vi "Server Cmd Parser - Set Corrections.vi"(8 "error in":errorcluster, 10 "client request":T1={"info data"="", "answer handle"=-1}, 11 "session in":T2={"adc"={"niScope"={"channel cfg"=[], "sessions"=[], "multi cards"=FALSE, "channels"=0, "type"=enum."n/a", "memory [B/chn]"=0, "ext. clock [Hz]"=0.0, "samples count"=0, "use streaming"=FALSE, "proc setup"={"packet size [smpl]"=0, "current timeout [s]"=0.0, "blk2blk timeout [s]"=0.0, "event time"=timestamp(0 s since 1904-01-01), "temp sampl T [s]"=0.0, "data queue"=refnum, "stop notifier"=refnum, "proc ref"=refnum}, "sample width [B]"=0, "ranges [V]"=[], "trigger setup"={"coupling"=1, "level [V]"=0.0, "slope"=0, "mode"=enum."Immediate"}, "fs [Hz]"=0.0, "bitres [bit]"=0}, "3458A"={"channels"=[], "sync unit"={"VISA"="", "type"=enum."Picotest U6200A"}, "awg unit"={"type"=enum."Agilent 331xxA to 332xxA", "VISA"="", "enable 10MHz ref"=FALSE}, "sync mode"=enum."MASTER-SLAVE, MASTER clocked by TIMER", "streaming mode"=FALSE, "idn mode"=enum."Auto", "sampling mode"=enum."DCV", "Ts [s]"=0.0, "sample memory [B]"=0, "proc setup"={"channel id"=0, "packet size [smpl]"=0, "current timeout [s]"=0.0, "blk2blk timeout [s]"=0.0, "event time"=timestamp(0 s since 1904-01-01), "stop notifier"=refnum, "data queues"=[], "proc refs"=[], "bus semaphore"=refnum}, "sample size [B]"=0, "sample count"=0, "aux data"={"channel id"=0, "valid?"=[], "gain [V]"=[], "timestamp [s]"=[], "Ts [s]"=0.0, "abs timestamp"=timestamp(0 s since 1904-01-01), "t [deg C]"=[]}, "ranges [V]"=[], "aperture [s]"=0.0, "LEVEL trigger"={"edge"=enum."POS", "level [V]"=0.0, "coupling"=enum."DC"}, "trigger mode"=enum."AUTO", "measure temp.?"=FALSE, "disp mesages"=[], "shared bus?"=FALSE, "disable display?"=FALSE, "aper mode"=enum."Manual", "aper rules"=[]}, "dsdll"={"dsdll"={"dsdll path"=path "", "dsdll handle"=[], "output devices"=[], "capture devices"=[]}, "channels"=0, "device id"=0, "channel idns"=[], "proc setup"={"packet size [smpl]"=0, "current timeout [s]"=0.0, "blk2blk timeout [s]"=0.0, "event time"=timestamp(0 s since 1904-01-01), "data queue"=refnum, "stop notifier"=refnum, "proc ref"=refnum}, "samples count"=0, "fs [Hz]"=0.0}, "type"=enum."niScope", "channel idn str"=[], "aux instr idn str"=[], "modified?"=FALSE, "simadc"={"channels"=[], "range [V]"=0.0, "Ts step [s]"=0.0, "time [s]"=0.0, "fs [Hz]"=0.0, "count"=0, "smpl offset"=0, "set count"=0, "bit res"=0}, "force rst?"=FALSE, "exit mode"=enum."Immediate reset", "exit dly"=0.0, "exit tmr"=timestamp(0 s since 1904-01-01), "busy?"=FALSE, "accessed?"=FALSE, "QuADC session"={"channel cfg"=[], "sessions"=[], "multi cards"=FALSE, "channels"=0, "type"=enum."n/a", "memory [B/chn]"=0, "ext. clock [Hz]"=0.0, "samples count"=0, "use streaming"=FALSE, "proc setup"={"packet size [smpl]"=0, "current timeout [s]"=0.0, "blk2blk timeout [s]"=0.0, "event time"=timestamp(0 s since 1904-01-01), "temp sampl T [s]"=0.0, "data queue"=refnum, "stop notifier"=refnum, "proc ref"=refnum}, "sample width [B]"=0, "ranges [V]"=[], "trigger setup"={"coupling"=1, "level [V]"=0.0, "slope"=0, "mode"=enum."Immediate"}, "fs [Hz]"=0.0, "bitres [bit]"=0}}, "sequence"=[], "sequence setup"={"group setups"=[], "average cycles"=0, "range mode"=enum."Keep defaults", "fs mode"=enum."Frequency", "rng even"=0.0, "rng odd"=0.0, "folder"=path "", "name base"="", "meas id"=0, "settle [s]"=0.0}, "golpi"=refnum, "processing setup"={"mode"=enum."Raw", "call after avgs?"=FALSE, "calculate?"=FALSE, "raw mode"={"command"="", "result mode"=enum."Display console output (only Octave)", "res variable"=""}, "QWTB"={"QWTB path"=path "", "alg filter path"="", "alg ids"=[], "alg parameters"=[], "parsed parameters"=[], "selected alg id"="", "selected unc mode"=enum."None", "qwtb mcc"=100, "qwtb timeout"=90, "qwtb covg"=95.0, "qwtb ofs"=0, "qwtb lim data"=0, "multicore"={"jobs folder"=path "", "cores"=0, "max jobs"=0, "mode"=enum."Singlecore"}, "unc once?"=FALSE}}, "corrections"={"transducers"={"channels"=[], "last path"=path ""}, "digitizer"={"last path"=path "", "channel paths"=[], "channel idns"=[], "correction name"="", "channel names"=[], "folders to copy"=[], "channel valid"=[], "correction path"=path "", "correction rel path"="", "rel folders to copy"=[]}}, "assist cfg"={"P"=0, "Q"=0, "rel shift"=0.0, "ref freq"=0.0, "min fs"=0.0, "max fs tol"=0.0, "min int"=0.0, "max int"=0.0, "max err"=0.0, "max timeout"=0.0}} {"corrections"."transducers"."channels"."Phase index" min=1 step=1; "adc"."QuADC session"."trigger setup"."level [V]" format="%.2f"; "adc"."QuADC session"."trigger setup"."coupling" items=["AC"=0, "DC"=1, "HF Reject"=3, "LF Reject"=4, "AC Plus HF Reject"=1001]; "adc"."QuADC session"."channel cfg"."Clock fr. (Hz)" min=0.0 format="%#_9p"; "adc"."QuADC session"."channel cfg"."Number of JJ" min=1; "adc"."QuADC session"."channel cfg"."Range [Vpk]" min=0.0; "adc"."QuADC session"."channel cfg"."Channel" min=0; "adc"."3458A"."channels"."Range [Vpk]" min=0.0; "adc"."niScope"."trigger setup"."level [V]" format="%.2f"; "adc"."niScope"."trigger setup"."coupling" items=["AC"=0, "DC"=1, "HF Reject"=3, "LF Reject"=4, "AC Plus HF Reject"=1001]; "adc"."niScope"."channel cfg"."Range [Vpk]" min=0.0; "adc"."niScope"."channel cfg"."Channel" min=0}) -> (0 "error out":errorcluster, 3 "session out":T2={"adc"={"niScope"={"channel cfg"=[], "sessions"=[], "multi cards"=FALSE, "channels"=0, "type"=enum."n/a", "memory [B/chn]"=0, "ext. clock [Hz]"=0.0, "samples count"=0, "use streaming"=FALSE, "proc setup"={"packet size [smpl]"=0, "current timeout [s]"=0.0, "blk2blk timeout [s]"=0.0, "event time"=timestamp(0 s since 1904-01-01), "temp sampl T [s]"=0.0, "data queue"=refnum, "stop notifier"=refnum, "proc ref"=refnum}, "sample width [B]"=0, "ranges [V]"=[], "trigger setup"={"coupling"=1, "level [V]"=0.0, "slope"=0, "mode"=enum."Immediate"}, "fs [Hz]"=0.0, "bitres [bit]"=0}, "3458A"={"channels"=[], "sync unit"={"VISA"="", "type"=enum."Picotest U6200A"}, "awg unit"={"type"=enum."Agilent 331xxA to 332xxA", "VISA"="", "enable 10MHz ref"=FALSE}, "sync mode"=enum."MASTER-SLAVE, MASTER clocked by TIMER", "streaming mode"=FALSE, "idn mode"=enum."Auto", "sampling mode"=enum."DCV", "Ts [s]"=0.0, "sample memory [B]"=0, "proc setup"={"channel id"=0, "packet size [smpl]"=0, "current timeout [s]"=0.0, "blk2blk timeout [s]"=0.0, "event time"=timestamp(0 s since 1904-01-01), "stop notifier"=refnum, "data queues"=[], "proc refs"=[], "bus semaphore"=refnum}, "sample size [B]"=0, "sample count"=0, "aux data"={"channel id"=0, "valid?"=[], "gain [V]"=[], "timestamp [s]"=[], "Ts [s]"=0.0, "abs timestamp"=timestamp(0 s since 1904-01-01), "t [deg C]"=[]}, "ranges [V]"=[], "aperture [s]"=0.0, "LEVEL trigger"={"edge"=enum."POS", "level [V]"=0.0, "coupling"=enum."DC"}, "trigger mode"=enum."AUTO", "measure temp.?"=FALSE, "disp mesages"=[], "shared bus?"=FALSE, "disable display?"=FALSE, "aper mode"=enum."Manual", "aper rules"=[]}, "dsdll"={"dsdll"={"dsdll path"=path "", "dsdll handle"=[], "output devices"=[], "capture devices"=[]}, "channels"=0, "device id"=0, "channel idns"=[], "proc setup"={"packet size [smpl]"=0, "current timeout [s]"=0.0, "blk2blk timeout [s]"=0.0, "event time"=timestamp(0 s since 1904-01-01), "data queue"=refnum, "stop notifier"=refnum, "proc ref"=refnum}, "samples count"=0, "fs [Hz]"=0.0}, "type"=enum."niScope", "channel idn str"=[], "aux instr idn str"=[], "modified?"=FALSE, "simadc"={"channels"=[], "range [V]"=0.0, "Ts step [s]"=0.0, "time [s]"=0.0, "fs [Hz]"=0.0, "count"=0, "smpl offset"=0, "set count"=0, "bit res"=0}, "force rst?"=FALSE, "exit mode"=enum."Immediate reset", "exit dly"=0.0, "exit tmr"=timestamp(0 s since 1904-01-01), "busy?"=FALSE, "accessed?"=FALSE, "QuADC session"={"channel cfg"=[], "sessions"=[], "multi cards"=FALSE, "channels"=0, "type"=enum."n/a", "memory [B/chn]"=0, "ext. clock [Hz]"=0.0, "samples count"=0, "use streaming"=FALSE, "proc setup"={"packet size [smpl]"=0, "current timeout [s]"=0.0, "blk2blk timeout [s]"=0.0, "event time"=timestamp(0 s since 1904-01-01), "temp sampl T [s]"=0.0, "data queue"=refnum, "stop notifier"=refnum, "proc ref"=refnum}, "sample width [B]"=0, "ranges [V]"=[], "trigger setup"={"coupling"=1, "level [V]"=0.0, "slope"=0, "mode"=enum."Immediate"}, "fs [Hz]"=0.0, "bitres [bit]"=0}}, "sequence"=[], "sequence setup"={"group setups"=[], "average cycles"=0, "range mode"=enum."Keep defaults", "fs mode"=enum."Frequency", "rng even"=0.0, "rng odd"=0.0, "folder"=path "", "name base"="", "meas id"=0, "settle [s]"=0.0}, "golpi"=refnum, "processing setup"={"mode"=enum."Raw", "call after avgs?"=FALSE, "calculate?"=FALSE, "raw mode"={"command"="", "result mode"=enum."Display console output (only Octave)", "res variable"=""}, "QWTB"={"QWTB path"=path "", "alg filter path"="", "alg ids"=[], "alg parameters"=[], "parsed parameters"=[], "selected alg id"="", "selected unc mode"=enum."None", "qwtb mcc"=100, "qwtb timeout"=90, "qwtb covg"=95.0, "qwtb ofs"=0, "qwtb lim data"=0, "multicore"={"jobs folder"=path "", "cores"=0, "max jobs"=0, "mode"=enum."Singlecore"}, "unc once?"=FALSE}}, "corrections"={"transducers"={"channels"=[], "last path"=path ""}, "digitizer"={"last path"=path "", "channel paths"=[], "channel idns"=[], "correction name"="", "channel names"=[], "folders to copy"=[], "channel valid"=[], "correction path"=path "", "correction rel path"="", "rel folders to copy"=[]}}, "assist cfg"={"P"=0, "Q"=0, "rel shift"=0.0, "ref freq"=0.0, "min fs"=0.0, "max fs tol"=0.0, "min int"=0.0, "max int"=0.0, "max err"=0.0, "max timeout"=0.0}} {"corrections"."transducers"."channels"."Phase index" min=1 step=1; "adc"."QuADC session"."trigger setup"."level [V]" format="%.2f"; "adc"."QuADC session"."trigger setup"."coupling" items=["AC"=0, "DC"=1, "HF Reject"=3, "LF Reject"=4, "AC Plus HF Reject"=1001]; "adc"."QuADC session"."channel cfg"."Clock fr. (Hz)" min=0.0 format="%#_9p"; "adc"."QuADC session"."channel cfg"."Number of JJ" min=1; "adc"."QuADC session"."channel cfg"."Range [Vpk]" min=0.0; "adc"."QuADC session"."channel cfg"."Channel" min=0; "adc"."3458A"."channels"."Range [Vpk]" min=0.0; "adc"."niScope"."trigger setup"."level [V]" format="%.2f"; "adc"."niScope"."trigger setup"."coupling" items=["AC"=0, "DC"=1, "HF Reject"=3, "LF Reject"=4, "AC Plus HF Reject"=1001]; "adc"."niScope"."channel cfg"."Range [Vpk]" min=0.0; "adc"."niScope"."channel cfg"."Channel" min=0})   [LabVIEW 2018]
doc: "Parses Server command \"Set corrections\" and assigns the parsed parameters to the measurement session."
uses:
  measure/Meas Session.ctl
  adc/ADC Session.ctl
  drivers/niScope/niScope Session.ctl
  drivers/niScope/niScope Virtual Channel Config.ctl
  drivers/niScope/niScope Virtual Channel Mode.ctl
  drivers/niScope/niScope Virtual Channel Input Z.ctl
  drivers/niScope/niScope Virtual Channel Coupling.ctl
  drivers/niScope/niScope Type.ctl
  drivers/niScope/niScope Digitizing Process Options.ctl
  drivers/niScope/niScope Data Packet.ctl
  drivers/niScope/niScope Trigger Setup.ctl
  <instrlib>/niScope/Controls/niScope trigger coupling.ctl
  <instrlib>/niScope/Controls/niScope trigger slope.ctl
  drivers/DMM/3458A Digitizer Session.ctl
  drivers/DMM/3458A Virtual Channel Config.ctl
  drivers/Counter/Counter Session.ctl
  drivers/Counter/Counter Type.ctl
  drivers/AWG/AWG Session.ctl
  drivers/AWG/AWG Type.ctl
  drivers/DMM/3458A Sync Mode.ctl
  drivers/DMM/3458A Idn Mode.ctl
  drivers/DMM/3458A Digitizing Low Levels/Configure/Sampling Mode.ctl
  drivers/DMM/3458A Digitizing Process Options.ctl
  drivers/DMM/3458A Data Packet.ctl
  drivers/DMM/3458A Aux Record Data.ctl
  drivers/DMM/3458A Digitizing Low Levels/Configure/Level Setup.ctl
  drivers/DMM/3458A Digitizing Low Levels/Configure/First Sample Trigger.ctl
  drivers/DMM/3458A Aperture Selection Mode.ctl
  drivers/dsdll/DSDLL Session.ctl
  drivers/dsdll/dsdll source distribution/dsdll_instance.ctl
  drivers/dsdll/dsdll source distribution/dsdll_device_record.ctl
  drivers/dsdll/DSDLL Process Config.ctl
  drivers/dsdll/DSDLL Data Packet.ctl
  adc/ADC Type.ctl
  drivers/simulated_adc/SimAdc Config.ctl
  drivers/simulated_adc/SimAdc Channel Cfg.ctl
  adc/ADC On Close Action.ctl
  drivers/Quatsch_driver/QuADCDriver/QuADC Session.ctl
  drivers/Quatsch_driver/QuADCDriver/QuADC Virtual Channel Config.ctl
  drivers/Quatsch_driver/QuADCDriver/QuADC Virtual Channel Mode.ctl
  drivers/Quatsch_driver/QuADCDriver/QuADC Virtual Channel Input Z.ctl
  drivers/Quatsch_driver/QuADCDriver/QuADC Virtual Channel Coupling.ctl
  drivers/Quatsch_driver/QuADCDriver/QuADC Type.ctl
  drivers/Quatsch_driver/QuADCDriver/QuADC Digitizing Process Options.ctl
  drivers/Quatsch_driver/QuADCDriver/QuADC Data Packet.ctl
  drivers/Quatsch_driver/QuADCDriver/QuADC Trigger Setup.ctl
  measure/Meas Sequence Item.ctl
  measure/Meas Sampling Configuration.ctl
  adc/ADC Trig Config.ctl
  adc/ADC Trig Mode Source.ctl
  adc/ADC Trig Coupling.ctl
  adc/ADC Trig Slope.ctl
  measure/processing/QWTB/Meas Proc QWTB Algorithm Parameter Data.ctl
  measure/Meas Sequence Configuration.ctl
  measure/Meas Range Mode.ctl
  measure/Meas Sampling Rate Mode.ctl
  octave/golpi/mpc/golpi_session_ref.ctl
  octave/golpi/mpc/golpi_session.ctl
  octave/golpi/GOLPI Library.lvlibp/Public/GOLPI reference Type Def.ctl
  octave/golpi/GOLPI Library.lvlibp/LV Process source distribution/Pipe Handle.ctl
  measure/processing/Meas Process Config.ctl
  measure/processing/Meas Process Mode.ctl
  measure/processing/Meas Process Raw Config.ctl
  measure/processing/Meas Process Raw Result Mode.ctl
  measure/processing/QWTB/Meas Proc QWTB Setup.ctl
  measure/processing/QWTB/Meas Proc QWTB Uncertainty Mode.ctl
  measure/processing/QWTB/Meas Proc QWTB Multicore Setup.ctl
  measure/processing/QWTB/Meas Proc QWTB Multicore Type.ctl
  measure/Corrections/Corr Setup.ctl
  measure/Corrections/Corr Tranducer Item.ctl
  measure/Corrections/Corr Digitizers.ctl
  measure/Assist/Assist Panel Setup.ctl
  Server Client Request.ctl
  octave/infolib.lvlibp/Private/Get matrix polymorph parts/Get 1D String.vi
  octave/infolib.lvlibp/Private/Get matrix polymorph parts/Get 1D I64.vi
  octave/infolib.lvlibp/Private/Get key polymorph parts/GetString.vi
  octave/infolib.lvlibp
  drivers/niScope/niScope Virtual Digitizer.lvlib
  drivers/DMM/3458A Virtual Digitizer.lvlib
  drivers/Counter/Counter.lvlib
  drivers/AWG/AWG.lvlib
  drivers/DMM/3458A Digitizing Low Levels/3458A Digitizing Low Levels.lvlib
  drivers/dsdll/DSDLL Virtual Digitizer.lvlib
  octave/golpi/GOLPI Library.lvlibp/LV Process source distribution/LV Process library.lvlib
  octave/golpi/GOLPI Library.lvlibp
  octave/golpi/mpc/GOLPI Multi Process.lvlib
  drivers/Quatsch_driver/QuADCDriver/QuADC Virtual Digitizer.lvlib
  drivers/dsdll/dsdll source distribution/dsdll.lvlib
panel:
  # "ADC:"
  # "IP Address"
  # "."
  # "."
  # "."
  # ":"
  # "ADC:"
  # "IP Address"
  # "."
  # "."
  # "."
  # ":"
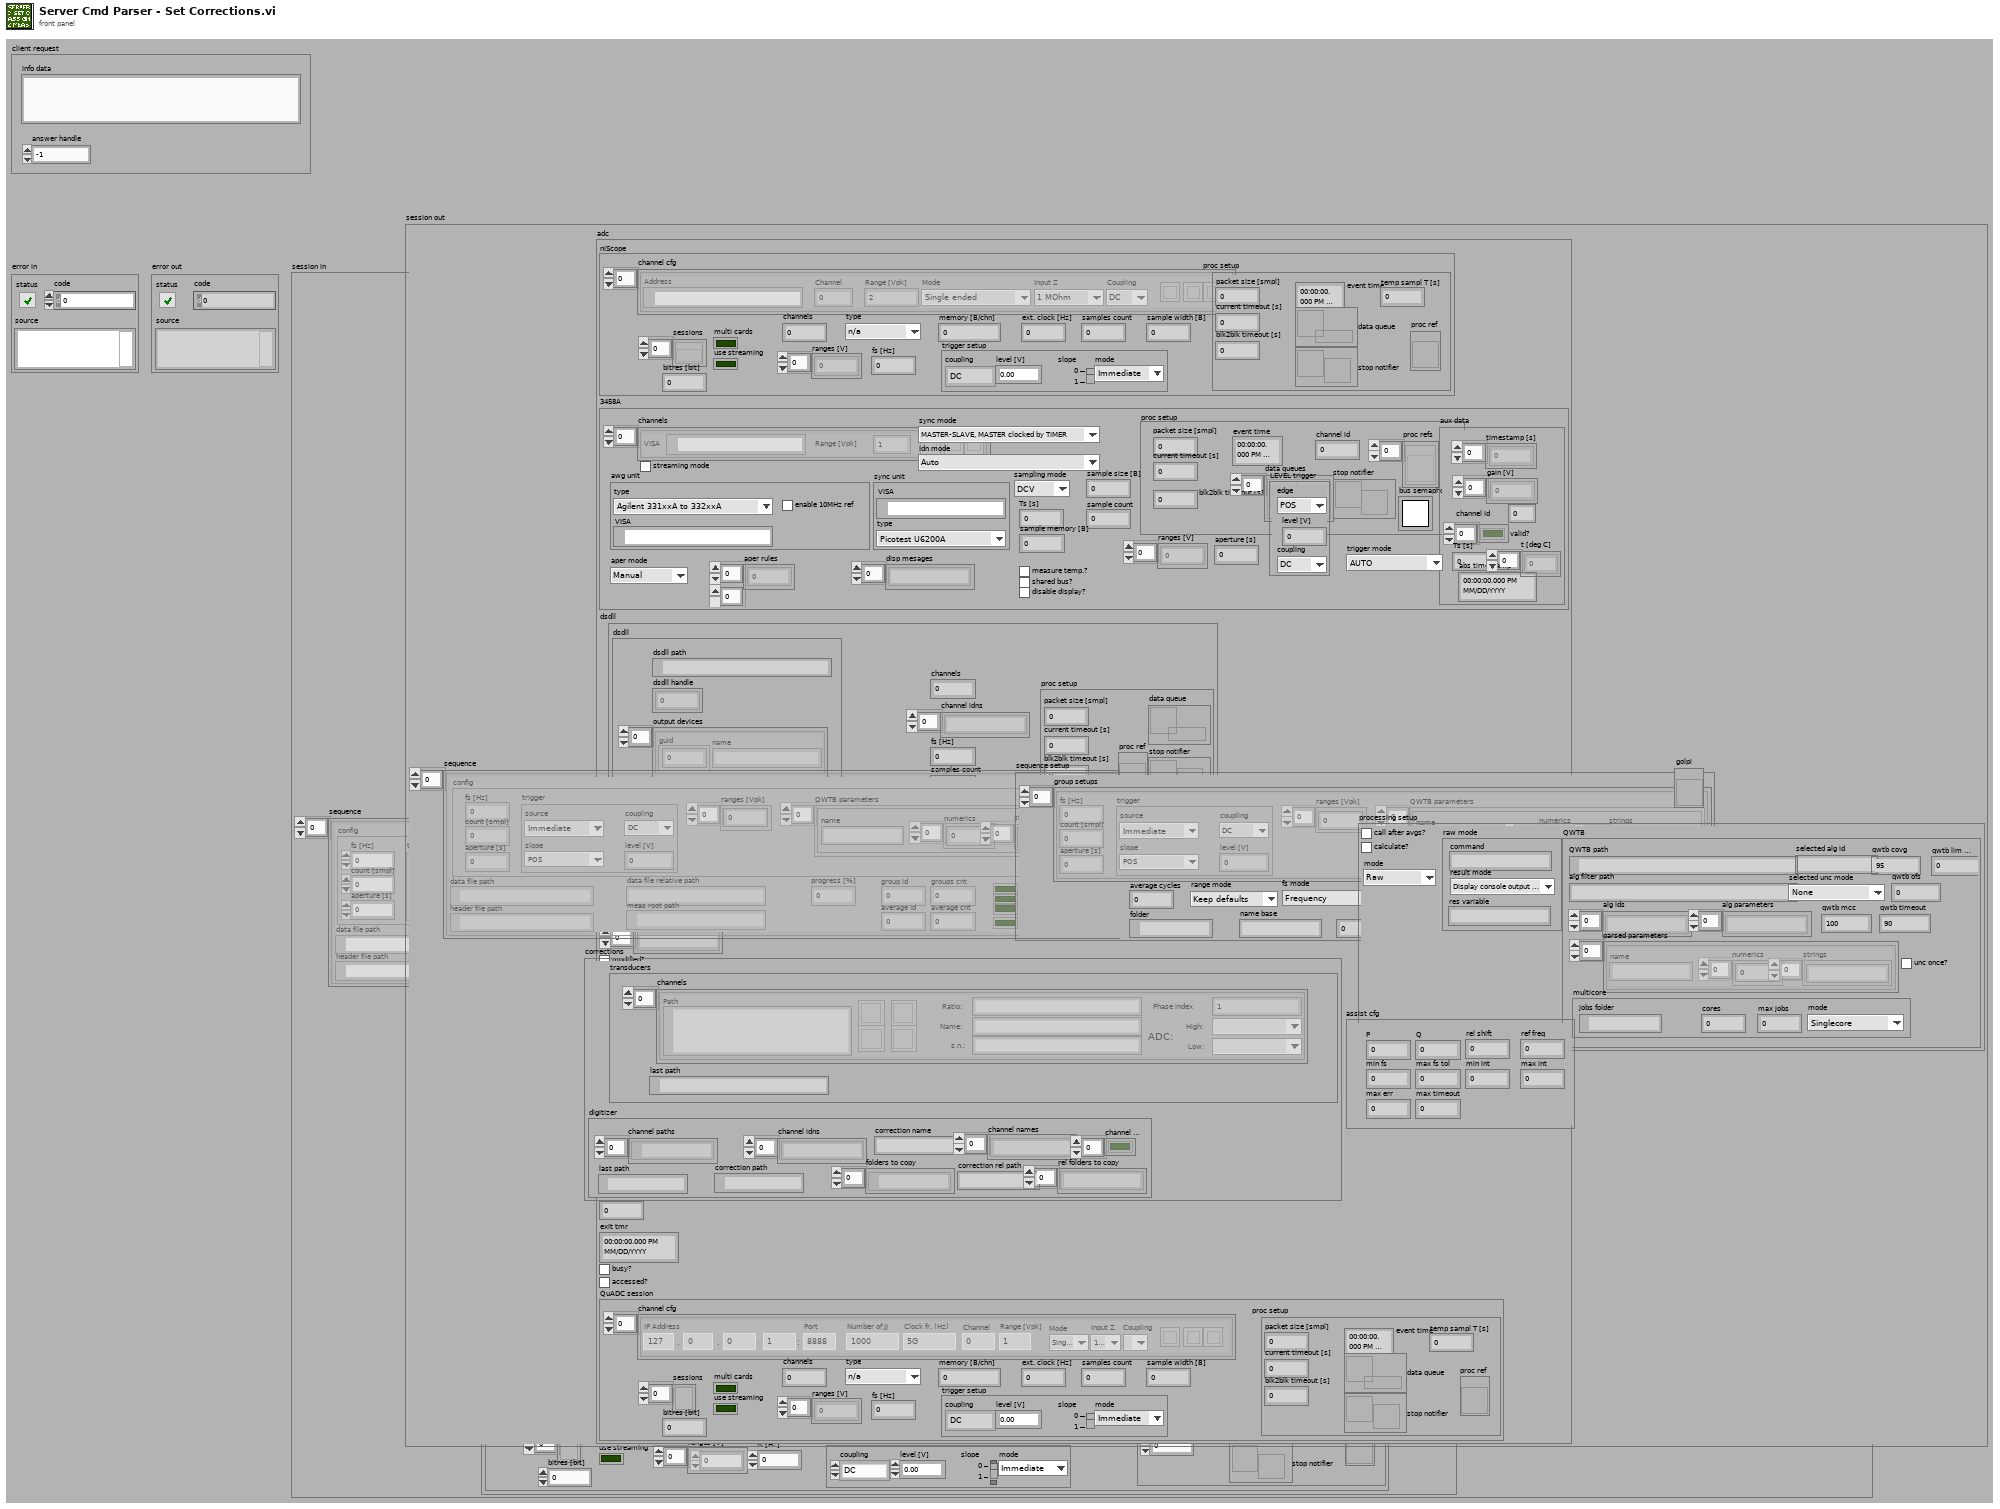
[diagram p1: front panel]
types:
  T1 = typedef "Server Client Request.ctl" = cluster{"info data":string, "answer handle":i32}
  T2 = typedef "Meas Session.ctl" = cluster{"adc":T3, "sequence":T45[], "sequence setup":T52, "golpi":T55, "processing setup":T56, "corrections":T64, "assist cfg":T67}
  T3 = typedef "ADC Session.ctl" = cluster{"niScope":T4, "3458A":T14, "dsdll":T29, "type":T33, "channel idn str":string[], "aux instr idn str":string[], "modified?":bool, "simadc":T34, "force rst?":bool, "exit mode":T36, "exit dly":dbl, "exit tmr":timestamp, "busy?":bool, "accessed?":bool, "QuADC session":T37}
  T4 = typedef "niScope Virtual Digitizer.lvlib/niScope Session.ctl" = cluster{"channel cfg":T5[], "sessions":refnum<k20>[], "multi cards":bool, "channels":i32, "type":T9, "memory [B/chn]":i32, "ext. clock [Hz]":dbl, "samples count":i64, "use streaming":bool, "proc setup":T10, "sample width [B]":i32, "ranges [V]":dbl[], "trigger setup":T11, "fs [Hz]":dbl, "bitres [bit]":i32}
  T5 = typedef "niScope Virtual Digitizer.lvlib/niScope Virtual Channel Config.ctl" = cluster{"Address":refnum<k15>, "Channel":i32, "Mode":T6, "Input Z":T7, "Coupling":T8, "Range [Vpk]":dbl, "btn clr":bool, "btn up":bool, "btn down":bool}
  T6 = typedef "niScope Virtual Digitizer.lvlib/niScope Virtual Channel Mode.ctl" = enum16{"Single ended", "Unbal. differential", "Differential"}
  T7 = typedef "niScope Virtual Digitizer.lvlib/niScope Virtual Channel Input Z.ctl" = enum16{"1 MOhm", "50 Ohm"}
  T8 = typedef "niScope Virtual Digitizer.lvlib/niScope Virtual Channel Coupling.ctl" = enum16{"AC", "DC", "GND"}
  T9 = typedef "niScope Virtual Digitizer.lvlib/niScope Type.ctl" = enum16{"n/a", "5922"}
  T10 = typedef "niScope Virtual Digitizer.lvlib/niScope Digitizing Process Options.ctl" = cluster{"packet size [smpl]":i64, "current timeout [s]":dbl, "blk2blk timeout [s]":dbl, "event time":timestamp, "temp sampl T [s]":dbl, "data queue":refnum<queue>, "stop notifier":refnum<notifier>, "proc ref":refnum<vi>}
  T11 = typedef "niScope Virtual Digitizer.lvlib/niScope Trigger Setup.ctl" = cluster{"coupling":T12, "level [V]":dbl, "slope":T13, "mode":enum16{"Immediate", "External", "Level"}}
  T12 = typedef "niScope trigger coupling.ctl" = u16
  T13 = typedef "niScope trigger slope.ctl" = i32
  T14 = typedef "3458A Virtual Digitizer.lvlib/3458A Digitizer Session.ctl" = cluster{"channels":T15[], "sync unit":T16, "awg unit":T18, "sync mode":T20, "streaming mode":bool, "idn mode":T21, "sampling mode":T22, "Ts [s]":dbl, "sample memory [B]":i32, "proc setup":T23, "sample size [B]":i32, "sample count":i32, "aux data":T25, "ranges [V]":dbl[], "aperture [s]":dbl, "LEVEL trigger":T26, "trigger mode":T27, "measure temp.?":bool, "disp mesages":string[], "shared bus?":bool, "disable display?":bool, "aper mode":T28, "aper rules":dbl[][]}
  T15 = typedef "3458A Virtual Digitizer.lvlib/3458A Virtual Channel Config.ctl" = cluster{"VISA":refnum<visa-resource-name>, "Range [Vpk]":dbl, "btn clr":bool, "btn up":bool, "btn down":bool}
  T16 = typedef "Counter.lvlib/Counter Session.ctl" = cluster{"VISA":refnum<visa-resource-name>, "type":T17}
  T17 = typedef "Counter.lvlib/Counter Type.ctl" = enum16{"Picotest U6200A", "dummy"}
  T18 = typedef "AWG.lvlib/AWG Session.ctl" = cluster{"type":T19, "VISA":refnum<visa-resource-name>, "enable 10MHz ref":bool}
  T19 = typedef "AWG.lvlib/AWG Type.ctl" = enum16{"Agilent 331xxA to 332xxA", "Agilent 335xxA to 336xxA", "Tektronix AFG3101C", "dummy"}
  T20 = typedef "3458A Virtual Digitizer.lvlib/3458A Sync Mode.ctl" = enum16{"MASTER-SLAVE, MASTER clocked by TIMER", "MASTER-SLAVE, MASTER clocked by AWG", "ALL clocked by AWG", "MASTER-SLAVE, ALL clocked by TIMER", "ALL clocked by AWG with DFLL"}
  T21 = typedef "3458A Virtual Digitizer.lvlib/3458A Idn Mode.ctl" = enum16{"Auto", "Sequential (chn A, chn B, ...)", "From calibration string"}
  T22 = typedef "3458A Virtual Digitizer.lvlib/3458A Digitizing Low Levels.lvlib/Sampling Mode.ctl" = enum16{"DCV", "DSDC", "DSAC"}
  T23 = typedef "3458A Virtual Digitizer.lvlib/3458A Digitizing Process Options.ctl" = cluster{"channel id":i32, "packet size [smpl]":i32, "current timeout [s]":dbl, "blk2blk timeout [s]":dbl, "event time":timestamp, "stop notifier":refnum<notifier>, "data queues":refnum<queue>[], "proc refs":refnum<vi>[], "bus semaphore":T24}
  T24 = typedef "Semaphore RefNum" = refnum<k1>
  T25 = typedef "3458A Virtual Digitizer.lvlib/3458A Aux Record Data.ctl" = cluster{"channel id":i32, "valid?":bool[], "gain [V]":dbl[], "timestamp [s]":dbl[], "Ts [s]":dbl, "abs timestamp":timestamp, "t [deg C]":dbl[]}
  T26 = typedef "3458A Virtual Digitizer.lvlib/3458A Digitizing Low Levels.lvlib/Level Setup.ctl" = cluster{"edge":enum16{"POS", "NEG"}, "level [V]":dbl, "coupling":enum16{"DC", "AC"}}
  T27 = typedef "3458A Virtual Digitizer.lvlib/3458A Digitizing Low Levels.lvlib/First Sample Trigger.ctl" = enum16{"AUTO", "EXT", "SYN", "SGL", "HOLD", "LEVEL"}
  T28 = typedef "3458A Virtual Digitizer.lvlib/3458A Aperture Selection Mode.ctl" = enum16{"Manual", "Maximum", "Table"}
  T29 = typedef "DSDLL Virtual Digitizer.lvlib/DSDLL Session.ctl" = cluster{"dsdll":T30, "channels":i32, "device id":i32, "channel idns":string[], "proc setup":T32, "samples count":i32, "fs [Hz]":dbl}
  T30 = typedef "dsdll.lvlib/dsdll_instance.ctl" = cluster{"dsdll path":path, "dsdll handle":u8[], "output devices":T31[], "capture devices":T31[]}
  T31 = typedef "dsdll.lvlib/dsdll_device_record.ctl" = cluster{"guid":u8[], "name":string}
  T32 = typedef "DSDLL Virtual Digitizer.lvlib/DSDLL Process Config.ctl" = cluster{"packet size [smpl]":i32, "current timeout [s]":dbl, "blk2blk timeout [s]":dbl, "event time":timestamp, "data queue":refnum<queue>, "stop notifier":refnum<notifier>, "proc ref":refnum<vi>}
  T33 = typedef "ADC Type.ctl" = enum16{"niScope", "3458A", "DirectSound DLL", "dummy", "QuADC"}
  T34 = typedef "SimAdc Config.ctl" = cluster{"channels":T35[], "range [V]":dbl, "Ts step [s]":dbl, "time [s]":dbl, "fs [Hz]":dbl, "count":i64, "smpl offset":i64, "set count":i64, "bit res":i32}
  T35 = typedef "SimAdc Channel Cfg.ctl" = cluster{"harmonics":dbl[][], "btn clear":bool, "noise":dbl, "fundamental [Hz]":dbl}
  T36 = typedef "ADC On Close Action.ctl" = enum16{"Immediate reset", "Delayed reset"}
  T37 = typedef "QuADC Virtual Digitizer.lvlib/QuADC Session.ctl" = cluster{"channel cfg":T38[], "sessions":refnum<k5>[], "multi cards":bool, "channels":i32, "type":T42, "memory [B/chn]":i32, "ext. clock [Hz]":dbl, "samples count":i64, "use streaming":bool, "proc setup":T43, "sample width [B]":i32, "ranges [V]":dbl[], "trigger setup":T44, "fs [Hz]":dbl, "bitres [bit]":i32}
  T38 = typedef "QuADC Virtual Digitizer.lvlib/QuADC Virtual Channel Config.ctl" = cluster{"Channel":i32, "Mode":T39, "Input Z":T40, "Coupling":T41, "Range [Vpk]":dbl, "btn clr":bool, "btn up":bool, "btn down":bool, "IP address A":u8, "IP address B":u8, "IP address C":u8, "IP address D":u8, "Port":u16, "Number of JJ":u32, "Clock fr. (Hz)":dbl}
  T39 = typedef "QuADC Virtual Digitizer.lvlib/QuADC Virtual Channel Mode.ctl" = enum16{"Single ended", "Unbal. differential", "Differential"}
  T40 = typedef "QuADC Virtual Digitizer.lvlib/QuADC Virtual Channel Input Z.ctl" = enum16{"1 MOhm", "50 Ohm"}
  T41 = typedef "QuADC Virtual Digitizer.lvlib/QuADC Virtual Channel Coupling.ctl" = enum16{"AC", "DC", "GND"}
  T42 = typedef "QuADC Virtual Digitizer.lvlib/QuADC Type.ctl" = enum16{"n/a", "v1"}
  T43 = typedef "QuADC Virtual Digitizer.lvlib/QuADC Digitizing Process Options.ctl" = cluster{"packet size [smpl]":i64, "current timeout [s]":dbl, "blk2blk timeout [s]":dbl, "event time":timestamp, "temp sampl T [s]":dbl, "data queue":refnum<queue>, "stop notifier":refnum<notifier>, "proc ref":refnum<vi>}
  T44 = typedef "QuADC Virtual Digitizer.lvlib/QuADC Trigger Setup.ctl" = cluster{"coupling":T12, "level [V]":dbl, "slope":T13, "mode":enum16{"Immediate", "External", "Level"}}
  T45 = typedef "Meas Sequence Item.ctl" = cluster{"config":T46, "data file path":path, "header file path":path, "group id":i32, "average id":i32, "group done?":bool, "adc modified?":bool, "source modified?":bool, "progress [%]":dbl, "groups cnt":i32, "average cnt":i32, "data file relative path":string, "meas root path":path, "calculate?":bool}
  T46 = typedef "Meas Sampling Configuration.ctl" = cluster{"fs [Hz]":dbl, "count [smpl]":i64, "aperture [s]":dbl, "trigger":T47, "ranges [Vpk]":dbl[], "QWTB parameters":T51[]}
  T47 = typedef "ADC Trig Config.ctl" = cluster{"source":T48, "level [V]":dbl, "coupling":T49, "slope":T50}
  T48 = typedef "ADC Trig Mode Source.ctl" = enum16{"Immediate", "External", "Level"}
  T49 = typedef "ADC Trig Coupling.ctl" = enum16{"DC", "AC"}
  T50 = typedef "ADC Trig Slope.ctl" = enum16{"POS", "NEG"}
  T51 = typedef "Meas Proc QWTB Algorithm Parameter Data.ctl" = cluster{"name":string, "numerics":dbl[], "strings":string[]}
  T52 = typedef "Meas Sequence Configuration.ctl" = cluster{"group setups":T46[], "average cycles":i32, "range mode":T53, "fs mode":T54, "rng even":dbl, "rng odd":dbl, "folder":path, "name base":string, "meas id":i32, "settle [s]":dbl}
  T53 = typedef "Meas Range Mode.ctl" = enum16{"Keep defaults", "Set All channels", "Set Odd and Even channels"}
  T54 = typedef "Meas Sampling Rate Mode.ctl" = enum16{"Frequency", "Period"}
  T55 = typedef "GOLPI Multi Process.lvlib/golpi_session_ref.ctl" = refnum<vi>
  T56 = typedef "Meas Process Config.ctl" = cluster{"mode":T57, "call after avgs?":bool, "calculate?":bool, "raw mode":T58, "QWTB":T60}
  T57 = typedef "Meas Process Mode.ctl" = enum16{"Raw", "QWTB"}
  T58 = typedef "Meas Process Raw Config.ctl" = cluster{"command":string, "result mode":T59, "res variable":string}
  T59 = typedef "Meas Process Raw Result Mode.ctl" = enum16{"Display console output (only Octave)", "Display string variable", "Display result file %respath%"}
  T60 = typedef "Meas Proc QWTB Setup.ctl" = cluster{"QWTB path":path, "alg filter path":string, "alg ids":string[], "alg parameters":string[], "parsed parameters":T51[], "selected alg id":string, "selected unc mode":T61, "qwtb mcc":i32, "qwtb timeout":i32, "qwtb covg":dbl, "qwtb ofs":i64, "qwtb lim data":i64, "multicore":T62, "unc once?":bool}
  T61 = typedef "Meas Proc QWTB Uncertainty Mode.ctl" = enum16{"None", "GUF", "Monte Carlo"}
  T62 = typedef "Meas Proc QWTB Multicore Setup.ctl" = cluster{"jobs folder":path, "cores":i32, "max jobs":i32, "mode":T63}
  T63 = typedef "Meas Proc QWTB Multicore Type.ctl" = enum16{"Singlecore", "Multicore", "Multistation"}
  T64 = typedef "Corr Setup.ctl" = cluster{"transducers":cluster{"channels":T65[], "last path":path}, "digitizer":T66}
  T65 = typedef "Corr Tranducer Item.ctl" = cluster{"Path":path, "Ratio:":string, "Name:":string, "btn rem":bool, "btn up":bool, "btn down":bool, "s.n.:":string, "btn open":bool, "ratio o/i":dbl, "chn hi":u16, "chn lo":u16, "Phase index":i32}
  T66 = typedef "Corr Digitizers.ctl" = cluster{"last path":path, "channel paths":path[], "channel idns":string[], "correction name":string, "channel names":string[], "folders to copy":path[], "channel valid":bool[], "correction path":path, "correction rel path":string, "rel folders to copy":string[]}
  T67 = typedef "Assist Panel Setup.ctl" = cluster{"P":i32, "Q":i32, "rel shift":dbl, "ref freq":dbl, "min fs":dbl, "max fs tol":dbl, "min int":dbl, "max int":dbl, "max err":dbl, "max timeout":dbl}
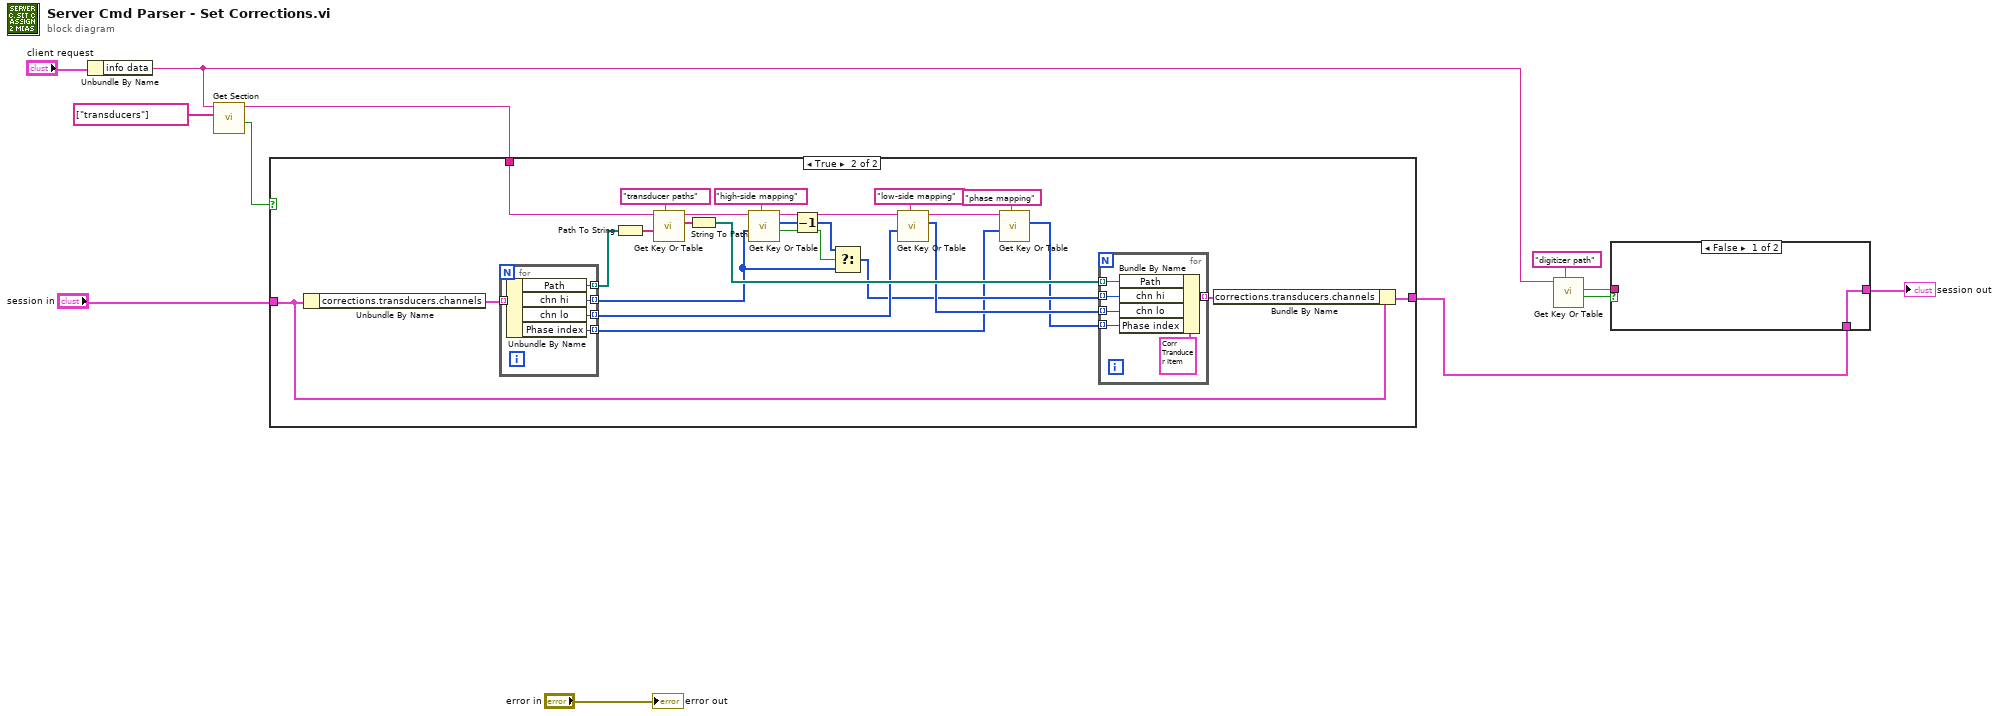
[diagram p0: block diagram]
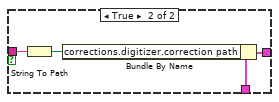
[diagram p2: hidden frame]
diagram:
  n1 = Unbundle By Name("client request") -> ("info data"=w5:string)
  n2 = call "Get Section.vi"("sections"=string[] ["transducers"], "info data"=w5) -> ("exist"=w7:bool, "section part"=w11:string)  [unwired: 8 in]
  n3 = case shown="True" w7 {
    tunnel: w11 -> [_ w33]
    tunnel: "session in" -> [w13 w26]
    tunnel: [w13 w25] -> w3
    frame False {
    }
    frame True {
      n4 = Unbundle By Name(w26) -> ("corrections.transducers.channels"=w27:T65[])
      n5 = for {
        tunnel: w27 -> [w49] mode=indexing
        tunnel: [w48] -> w32 mode=indexing
        tunnel: [w47] -> w19 mode=indexing
        tunnel: [w46] -> w24 mode=indexing
        tunnel: [w45] -> w15 mode=indexing
        n6 = Unbundle By Name(w49) -> ("Path"=w48:path, "chn hi"=w47:u16, "chn lo"=w46:u16, "Phase index"=w45:i32)
      }
      n7 = Path To String(path=w32) -> (string=w31:string[])
      n8 = call-poly "Get Key Or Table.vi"("key description"="transducer paths", "string"=w31, "info data"=w33) -> ("value"=w30:string[], "info data out"=w34:string)  [unwired: 5 in, 2 out]
      n9 = String To Path(string=w30) -> (path=w29:path[])
      n10 = call-poly "Get Key Or Table.vi"("key description"="high-side mapping", "numeric"=w19, "info data"=w34) -> ("found?"=w22:bool, "value"=w21:i64[], "info data out"=w36:string)  [unwired: 5 in, 1 out]
      n11 = Decrement(x=w21) -> (x-1=w18:i64[])
      n12 = Select(t=w18, s=w22, f=w19) -> (s? t:f=w20:i64[])
      n13 = call-poly "Get Key Or Table.vi"("key description"="low-side mapping", "numeric"=w24, "info data"=w36) -> ("value"=w23:i64[], "info data out"=w17:string)  [unwired: 5 in, 2 out]
      n14 = call-poly "Get Key Or Table.vi"("key description"="phase mapping", "numeric"=w15, "info data"=w17) -> ("value"=w14:i64[])  [unwired: 5 in, 3 out]
      n15 = for {
        tunnel: w29 -> [w43] mode=indexing
        tunnel: w23 -> [w42] mode=indexing
        tunnel: w20 -> [w41] mode=indexing
        tunnel: [w40] -> w28 mode=indexing
        tunnel: w14 -> [w39] mode=indexing
        n16 = Bundle By Name(cluster=T65 {"Path"=path "", "Ratio:"="", "Name:"="", "btn rem"=FALSE, "btn up"=FALSE, "btn down"=FALSE, "s.n.:"="", "btn open"=FALSE, "ratio o/i"=0.0, "chn hi"=0, "chn lo"=0, "Phase index"=1} ("Cluster"), "Path"=w43, "chn hi"=w41, "chn lo"=w42, "Phase index"=w39) -> (w40:T65)
      }
      n17 = Bundle By Name(cluster=w26, "corrections.transducers.channels"=w28) -> (w25:T2)
    }
  }
  n18 = call-poly "Get Key Or Table.vi"("key description"="digitizer path", "info data"=w5) -> ("found?"=w1:bool, "value"=w4:string)  [unwired: 6 in, 2 out]
  n19 = case shown="False" w1 {
    tunnel: w4 -> [_ w54]
    tunnel: w3 -> [w50 w53]
    tunnel: [w50 w51] -> w2
    frame False {
    }
    frame True {
      n20 = String To Path(string=w54) -> (path=w52:path)
      n21 = Bundle By Name(cluster=w53, "corrections.digitizer.correction path"=w52) -> (w51:T2)
    }
  }
  "session out" <- w2
  "error out" <- "error in"
